vi "EFW Get ID.vi"(8 "error in (no error)":errorcluster caption="错误输入（无错误）", 10 "ID":i32, 11 "index":i32) -> (0 "error out":errorcluster caption="错误输出", 2 "ID out":i32, 3 "function return":u32(ring))   [LabVIEW 2012, in "EFW_filter.lvlib"]
doc: "EFW_API EFW_ERROR_CODE EFWGetID(int index, int* ID);"
uses:
  <userlib>/EFW_filter/EFW_filter.lvlib
  <userlib>/EFW_filter/EFW_filter.dll
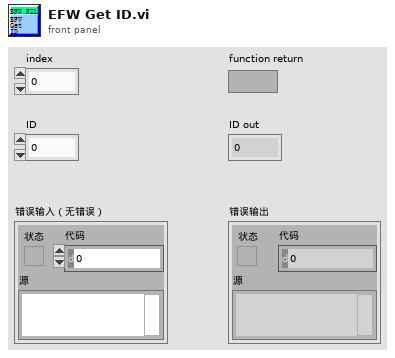
[diagram p1: front panel]
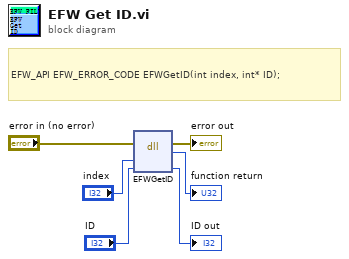
[diagram p0: block diagram]
diagram:
  # "EFW_API EFW_ERROR_CODE EFWGetID(int index, int* ID);"
  n1 = dll-call lib="D:/Program Files (x86)/National Instruments/LabVIEW 2012/user.lib/EFW_filter/EFW_filter.*" fn="EFWGetID"(error in="error in (no error)", "index"="index", "ID"="ID") -> (error out=→"error out":errorcluster, →"function return":u32, "ID"=→"ID out":i32)  [unwired: 3 in, 1 out]
